vi "CL3IF_GetMeasurementData.vi"(8 "error in":errorcluster {"code" format="%x"}, 11 "deviceId":i32) -> (0 "error out":errorcluster {"code" format="%x"}, 2 "MEASUREMENT_DATA":T1 caption="measurementData" {"outMeasurementData"."judgeResult" items=["HI"=1, "GO"=2, "LO"=4]})   [LabVIEW 2020, in "Keyence CL-3000.lvlib"]
doc: "This function gets the measurement values of all (eight) OUTs.\nThe measurement values of OUTs that have not been set are in judgment standby."
uses:
  Keyence CL-3000.lvlib
  clusters/CL3IF_MEASUREMENT_DATA.ctl
  clusters/CL3IF_OUTMEASUREMENT_DATA.ctl
  enums/CL3IF_VALUE_INFO.ctl
  enums/CL3IF_JUDGE_RESULT.ctl
  enums/CL3IF_OUTNO.ctl
  Private/enums/Function Name.ctl
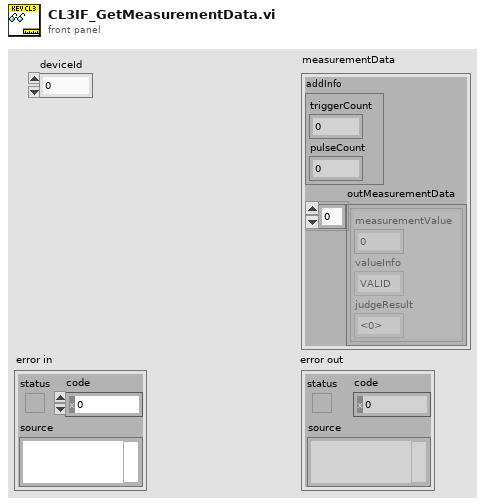
[diagram p1: front panel]
types:
  T1 = typedef "Keyence CL-3000.lvlib/CL3IF_MEASUREMENT_DATA.ctl" = cluster{"addInfo":cluster{"triggerCount":u32, "pulseCount":i32}, "outMeasurementData":T2[]}
  T2 = typedef "Keyence CL-3000.lvlib/CL3IF_OUTMEASUREMENT_DATA.ctl" = cluster{"measurementValue":i32, "valueInfo":T3, "judgeResult":T4}
  T3 = typedef "Keyence CL-3000.lvlib/CL3IF_VALUE_INFO.ctl" = enum8{"VALID", "JUDGMENTSTANDBY", "INVALID", "OVERDISPRANGE_P", "OVERDISPRANGE_N"}
  T4 = typedef "Keyence CL-3000.lvlib/CL3IF_JUDGE_RESULT.ctl" = u8
  T5 = typedef "Keyence CL-3000.lvlib/Function Name.ctl" = enum16{"Initialize", "Close", "CL3IF_GetMeasurementData", "CL3IF_GetTrendIndex", "CL3IF_GetTrendData", "CL3IF_GetStorageIndex", "CL3IF_GetStorageData", "CL3IF_AutoZeroMulti", "CL3IF_AutoZeroGroup", "CL3IF_TimingMulti", "CL3IF_TimingGroup", "CL3IF_ResetMulti", "CL3IF_ResetGroup", "CL3IF_LightControl", "CL3IF_MeasurementControl", "CL3IF_SwitchProgram", "CL3IF_GetProgramNo", "CL3IF_StartStorage", "CL3IF_StopStorage", "CL3IF_ClearStorageData", "CL3IF_GetPulseCount", "CL3IF_ResetPulseCount", "CL3IF_GetLightWaveform"}
  T6 = typedef "Keyence CL-3000.lvlib/CL3IF_OUTNO.ctl" = u16
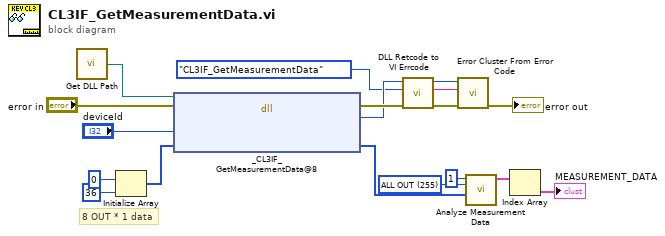
[diagram p0: block diagram]
diagram:
  w6 = T6 255 items=["OUT01"=1, "OUT02"=2, "OUT03"=4, "OUT04"=8, "OUT05"=16, "OUT06"=32, "OUT07"=64, "OUT08"=128, "ALL OUT"=255] ("outTarget")
  # "8 OUT * 1 data"
  n1 = call "Get DLL Path.vi"() -> ("DLL Path"=w14:path)  [unwired: 1 in]
  n2 = Initialize Array(u32 0, 36 ("x")) -> (w9:u32[])
  n3 = dll-call lib="C:/Program Files (x86)/National Instruments/LabVIEW 2018/instr.lib/Keyence CL-3000/CL3_IF.dll" fn="_CL3IF_GetMeasurementData@8"(path in=w14, error in="error in", "deviceid"="deviceId", "measurementData"=w9) -> (error out=w13:errorcluster, "RC"=w12:i32, "measurementData"=w8:u32[])  [unwired: 2 in, 1 out]
  n4 = call "DLL Retcode to VI Errcode.vi"("error in (no error)"=w13, "Function Name"=Function_Name."CL3IF_GetMeasurementData", "DLL Retcode"=w12) -> ("error out"=w18:errorcluster, "ErrorMessage"=w2:string, "VI Errcode"=w17:i32)  [unwired: 6 in]
  n5 = call <vilib>:"Error Cluster From Error Code.vi"("error in (no error)"=w18, "error message (\"\")"=w2, "error code (0)"=w17) -> ("error out"=→"error out":errorcluster)  [unwired: 6 in]
  n6 = call "Analyze Measurement Data.vi"("measurementData"=w8, "outTarget"=w6, "obtainedDataCount"=u32 1) -> ("MEASUREMENT_DATA"=w4:T1[])  [unwired: 8 in]
  n7 = Index Array(array=w4) -> (element=→"MEASUREMENT_DATA":T1)  [unwired: 1 in]
